vi "Signal who can eat.vi"(0 "Table in":refnum<class "Table.lvclass">, 11 "error in":errorcluster) -> (4 "Table out":refnum<class "Table.lvclass">, 15 "error out":errorcluster)   [LabVIEW 2023, in "Table.lvclass"]
uses:
  Table.lvclass
  C:/Program Files (x86)/National Instruments/LabVIEW 2023/vi.lib/addons/_Workers/Library/Classes/Worker/Worker.lvclass
  Table.lvclass/Table.ctl
  Fork.ctl
  Hungry.ctl
  <vilib>/addons/_Workers/Library/Classes/Message/Enqueue Message to Queue.vi
  <vilib>/addons/_Workers/Library/Classes/Message/Message.lvclass
  Philosopher/Philosopher.lvclass
  C:/Program Files (x86)/National Instruments/LabVIEW 2023/vi.lib/addons/_Workers/Library/Classes/Workers Object/Workers Object.lvclass
  C:/Projects/DPP Workers/Workers/Table/Table.lvclass
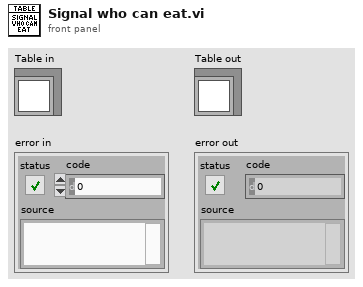
[diagram p1: front panel]
types:
  T1 = typedef "Table.lvclass/Hungry.ctl" = enum16{"NO", "YES"}
  T2 = typedef "Table.lvclass/Fork.ctl" = enum16{"FREE", "IN USE"}
  T3 = typedef "Workers.lvlib/Case Label.ctl" = string
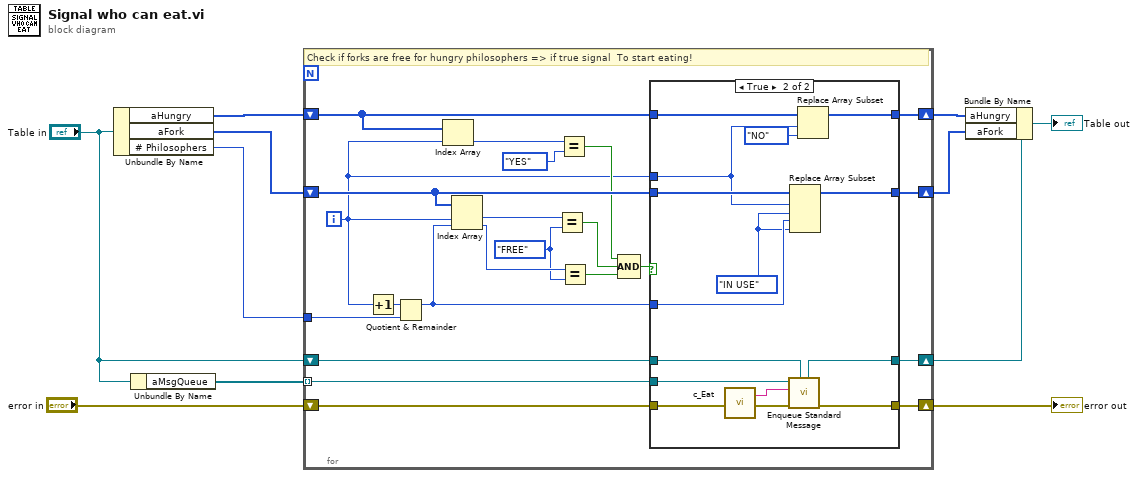
[diagram p0: block diagram]
diagram:
  n1 = Unbundle By Name("Table in") -> ("aHungry"=w11:T1[], "aFork"=w10:T2[], "# Philosophers"=w9:i32)
  n2 = Unbundle By Name("Table in") -> ("aMsgQueue"=w1:refnum<class "Message Queue.lvclass">[])
  n3 = for {
    tunnel: w9 -> [w32]
    shift-right: [w26] -> w5
    shift-left: w10 -> [w27]
    shift-right: [w22] -> w6
    shift-left: w11 -> [w23]
    shift-right: [w16] -> w8
    shift-left: "Table in" -> [w15]
    shift-right: [w13] -> w3
    shift-left: "error in" -> [w14]
    tunnel: w1 -> [w12] mode=indexing
    i -> [w21]
    w17 = Fork."FREE" ("y")
    # "Check if forks are free for hungry philosophers => if true signal  To start eating!"
    n4 = Increment(x=w21) -> (x+1=w33:i32)
    n5 = Quotient & Remainder(x=w33, y=w32) -> (x-y*floor(x/y)=w20:i32)  [unwired: 1 out]
    n6 = Index Array(array=w23, index=w21) -> (element=w25:T1)
    n7 = Index Array(array=w27, index #1=w21, index #2=w20) -> (element #1=w31:T2, element #2=w19:T2)
    n8 = Equal?(x=w31, y=w17) -> (x = y?=w29:bool)
    n9 = Equal?(x=w25, y=Hungry."YES") -> (x = y?=w24:bool)
    n10 = Equal?(x=w19, y=w17) -> (x = y?=w30:bool)
    n11 = Compound Arithmetic op=AND(w24, w29, w30) -> (w28:bool)
    n12 = case shown="True" w28 {
      tunnel: w27 -> [w37 w51]
      tunnel: w21 -> [_ w49]
      tunnel: w20 -> [_ w47]
      tunnel: [w37 w46] -> w26
      tunnel: w23 -> [w36 w50]
      tunnel: [w36 w48] -> w22
      tunnel: [w35 w43] -> w16
      tunnel: w15 -> [w35 w42]
      tunnel: w14 -> [w34 w40]
      tunnel: [w34 w39] -> w13
      tunnel: w12 -> [_ w38]
      frame False {
      }
      frame True {
        w44 = Fork."IN USE" ("new element/subarray")
        n13 = call "c_Eat.vi"() -> ("Case Label"=w41:T3)  [unwired: 1 in]
        n14 = call-poly <vilib>:"Enqueue Standard Message.vi"("Worker"=w42, "error in"=w40, "Case Label"=w41, "Message Queue"=w38) -> ("error out"=w39:errorcluster, "dup Worker out"=w43:refnum<class "Table.lvclass">)  [unwired: 5 in, 1 out]
        n15 = Replace Array Subset(array=w51, new element #1=w44, index #1=w49, new element #2=w44, index #2=w47) -> (w46:T2[])
        n16 = Replace Array Subset(array=w50, new element=Hungry."NO" ("new element/subarray"), index=w49) -> (w48:T1[])
      }
    }
  }
  "error out" <- w3
  n17 = Bundle By Name(cluster=w8, "aHungry"=w6, "aFork"=w5) -> (→"Table out":refnum<class "Table.lvclass">)
